vi "Formic Queen.vi"(8 "error in (no error)":errorcluster, 9 "SelfID":i32, 10 "Map":i32[](array[numeric]), 11 "Mother in":refnum<class "Mother.lvclass">) -> (0 "error out":errorcluster, 1 "Direction":T1, 2 "Action":T2, 3 "Mother out":refnum<class "Mother.lvclass">, 4 "Replicated Class":refnum<class "Mother.lvclass">)   [LabVIEW 2014, in "Mother.lvclass"]
uses:
  Mother.lvclass
  Action Enum.ctl
  Direction Enum.ctl
  Mother.lvclass/Mother.ctl
  SquareStatus.ctl
  Queen Bee Steps.ctl
  Formic Types.ctl
  SquareBattle.lvclass
panel:
  in  "Protectors":i32[](array[numeric])=[2, 6]
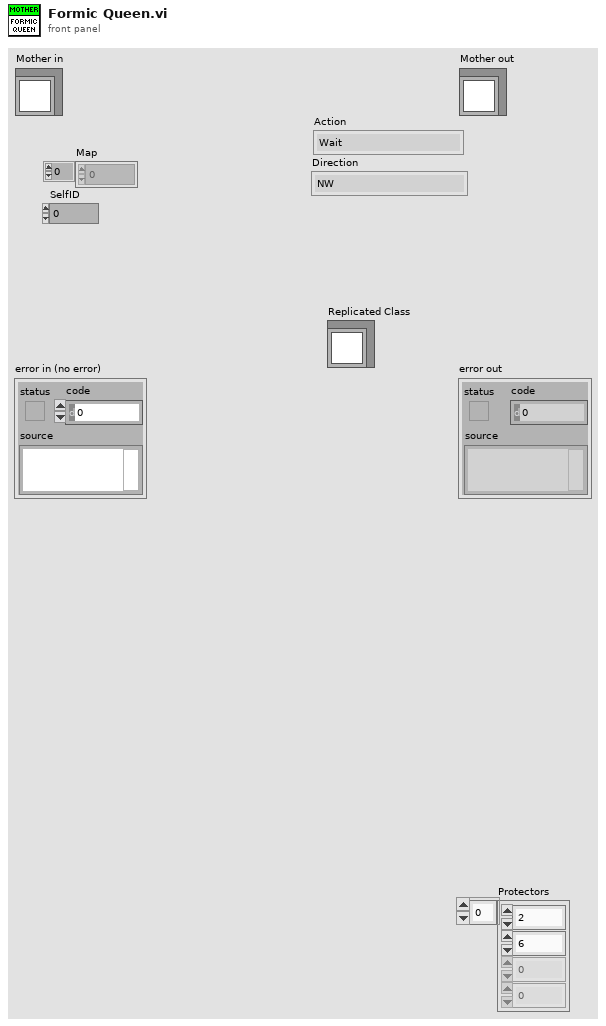
[diagram p1: front panel]
types:
  T1 = typedef "SquareBattle.lvclass/Direction Enum.ctl" = enum16{"NW", "N", "NE", "E", "SE", "S", "SW", "W"}
  T2 = typedef "SquareBattle.lvclass/Action Enum.ctl" = enum16{"Wait", "Move", "Attack", "Replicate"}
  T3 = typedef "Mother.lvclass/Formic Types.ctl" = enum16{"Queen Bee", "Protector Bee", "Daughter Bee", "Worker Bee", "Coward"}
  T4 = typedef "Mother.lvclass/SquareStatus.ctl" = cluster{"ID":i32, "Heartbeat":bool}
  T5 = typedef "Mother.lvclass/Queen Bee Steps.ctl" = enum16{"Attack?", "Migrate?", "Kamikaze?", "Protect?", "Procreate?", "Build Army"}
  T6 = typedef "Mother.lvclass/Kamikaze DVR.ctl" = refnum<data-value>
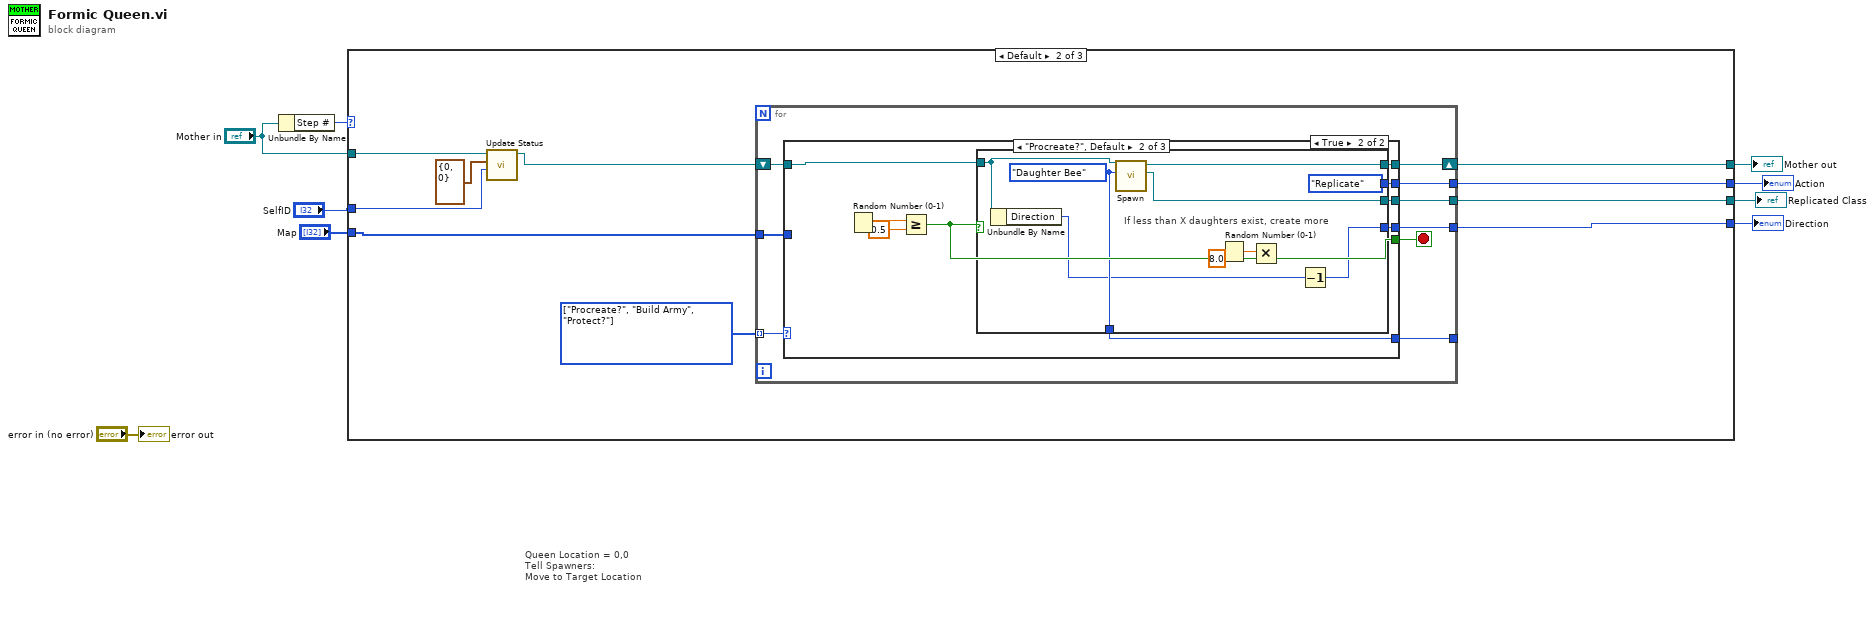
[diagram p0: block diagram]
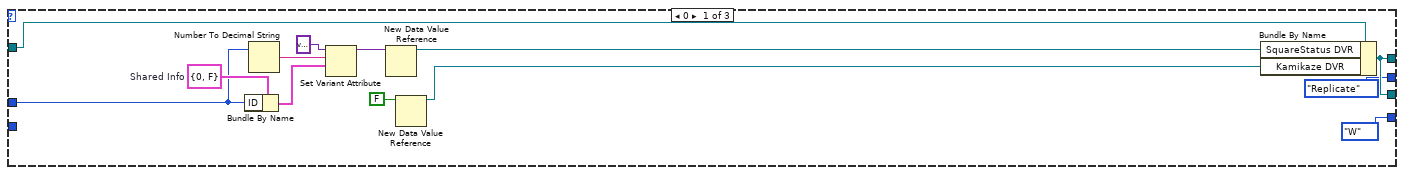
[diagram p2: hidden frame]
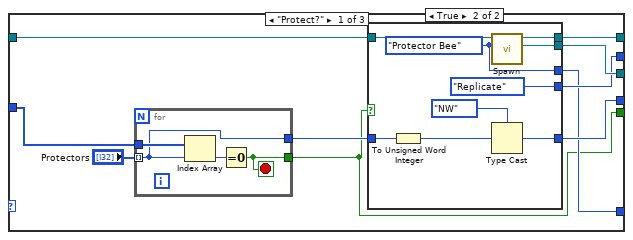
[diagram p3: hidden frame]
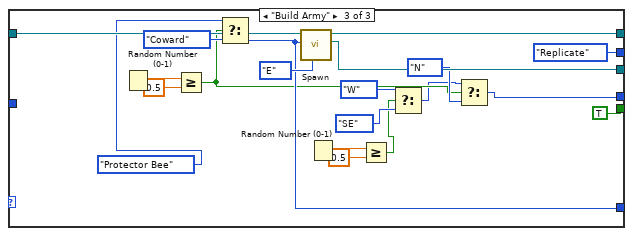
[diagram p6: hidden frame]
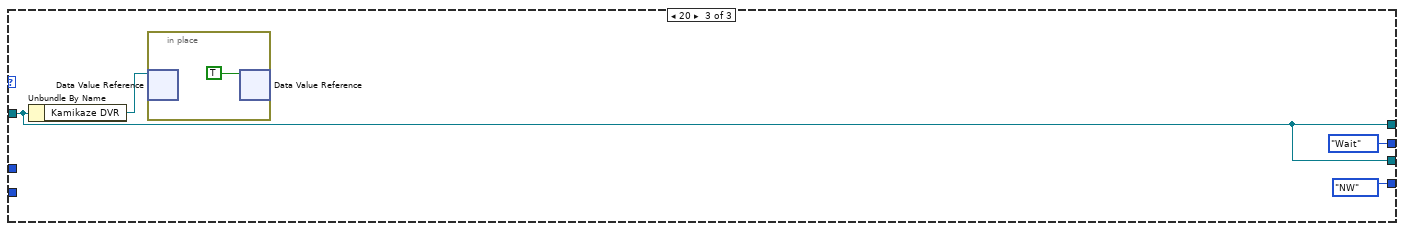
[diagram p7: hidden frame]
diagram:
  # "Queen Location = 0,0\nTell Spawners:\nMove to Target Location"
  n1 = Unbundle By Name("Mother in") -> ("Step #"=w6:i32)
  n2 = case shown="Default" w6 {
    tunnel: [w12 w28 w106] -> w8
    tunnel: "Mother in" -> [w14 w31 w106]
    tunnel: "SelfID" -> [w13 w30 _]
    tunnel: "Map" -> [_ w26 _]
    tunnel: [Action_Enum."Replicate" ("Action") w25 Action_Enum."Wait" ("Action")] -> w3
    tunnel: [Direction_Enum."W" ("Direction") w24 Direction_Enum."NW" ("Direction")] -> w2
    tunnel: [w12 w23 w106] -> w1
    frame 0 {
      w19 = T4 {"ID"=0, "Heartbeat"=FALSE}  # Shared Info
      n3 = Bundle By Name(cluster=w19, "ID"=w13) -> (w20:T4)
      n4 = Number To Decimal String(number=w13) -> (decimal integer string=w21:string)  [unwired: 1 in]
      n5 = Set Variant Attribute(Variant=variant ("variant"), name=w21, value=w20) -> (Variant out=w18:variant)  [unwired: 1 in, 2 out]
      n6 = New Data Value Reference(data value=w18) -> (data value reference=w17:refnum<data-value>)  [unwired: 1 in, 1 out]
      n7 = New Data Value Reference(data value=FALSE) -> (data value reference=w16:refnum<data-value>)  [unwired: 1 in, 1 out]
      n8 = Bundle By Name(cluster=w14, "SquareStatus DVR"=w17, "Kamikaze DVR"=w16) -> (w12:refnum<class "Mother.lvclass">)
    }
    frame Default {
      w27 = T5[] [enum."Procreate?", enum."Build Army", enum."Protect?"] items=["Attack?", "Migrate?", "Kamikaze?", "Protect?", "Procreate?", "Build Army"]
      n9 = call "Update Status.vi"("ID"=w30, "MyPosition"=cluster{"X":i32, "Y":i32} {"X"=0, "Y"=0}, "Mother in"=w31) -> ("Mother out"=w29:refnum<class "Mother.lvclass">)  [unwired: 8 in]
      n10 = for {
        shift-right: [w40] -> w28
        shift-left: w29 -> [w41]
        tunnel: [w39] -> w25
        tunnel: [w38] -> w24
        tunnel: w27 -> [w37] mode=indexing
        tunnel: [w35] -> w23
        tunnel: [w34] -> _
        tunnel: w26 -> [w33]
        stop <- w36 stop-if-true
        n11 = case shown="\"Procreate?\", Default" w37 {
          tunnel: w41 -> [w51 w69 w104]
          tunnel: [w50 w72 w101] -> w40
          tunnel: [w48 w74 Action_Enum."Replicate" ("Action")] -> w39
          tunnel: [w45 w73 w92] -> w38
          tunnel: [w43 w66 TRUE ("Enemy Found?")] -> w36
          tunnel: [w49 w71 w100] -> w35
          tunnel: [w44 w70 w94] -> w34
          tunnel: w33 -> [w42 _ _]
          frame "Protect?" {
            n12 = for {
              tunnel: w42 -> [w65]
              tunnel: [w64] -> w43
              tunnel: "Protectors" -> [w62] mode=indexing
              tunnel: [w62] -> w46
              stop <- w64 stop-if-true
              n13 = Index Array(array=w65, index=w62) -> (element=w63:i32)
              n14 = Equal To 0?(x=w63) -> (x = 0?=w64:bool)
            }
            n15 = case shown="True" w43 {
              tunnel: w51 -> [w52 w61]
              tunnel: [w52 w60] -> w50
              tunnel: [_ w59] -> w49
              tunnel: [_ Action_Enum."Replicate" ("Action")] -> w48
              tunnel: w46 -> [_ w56]
              tunnel: [_ w55] -> w45
              tunnel: [_ w53] -> w44
              frame False {
              }
              frame True {
                w53 = Formic_Types."Protector Bee"
                n16 = To Unsigned Word Integer(number=w56) -> (unsigned 16bit integer=w57:u16)
                n17 = call "Spawn.vi"(10:w53, "Mother in"=w61) -> ("Replicated Class"=w59:refnum<class "Mother.lvclass">, "Mother out"=w60:refnum<class "Mother.lvclass">)  [unwired: 7 in, 1 out]
                n18 = Type Cast(type=Direction_Enum."NW" ("Direction"), x=w57) -> (*(type *) &x=w55:T1)
              }
            }
          }
          frame "Procreate?", Default {
            n19 = Random Number (0-1)() -> (number: 0 to 1=w68:dbl)
            n20 = Greater Or Equal?(x=w68, y=0.5) -> (x >= y?=w66:bool)
            n21 = case shown="True" w66 {
              tunnel: [_ Action_Enum."Replicate" ("Action")] -> w74
              tunnel: [_ w78] -> w73
              tunnel: [w75 w83] -> w72
              tunnel: [_ w82] -> w71
              tunnel: [_ w81] -> w70
              tunnel: w69 -> [w75 w77]
              frame False {
              }
              frame True {
                w81 = Formic_Types."Daughter Bee"
                # "If less than X daughters exist, create more"
                n22 = Unbundle By Name(w77) -> ("Direction"=w76:T1)
                n23 = call "Spawn.vi"(10:w81, "Mother in"=w77) -> ("Replicated Class"=w82:refnum<class "Mother.lvclass">, "Mother out"=w83:refnum<class "Mother.lvclass">)  [unwired: 7 in, 1 out]
                n24 = Random Number (0-1)() -> (number: 0 to 1=w80:dbl)
                n25 = Multiply(x=w80, y=8.0) -> ()  [unwired: 1 out]
                n26 = Decrement(x=w76) -> (x-1=w78:T1)
              }
            }
          }
          frame "Build Army" {
            n27 = Random Number (0-1)() -> (number: 0 to 1=w95:dbl)
            n28 = Greater Or Equal?(x=w95, y=0.5) -> (x >= y?=w90:bool)
            n29 = Select(t=Formic_Types."Protector Bee", s=w90, f=Formic_Types."Coward") -> (s? t:f=w94:T3)
            n30 = call "Spawn.vi"("Start Direction"=Direction_Enum."E", 10:w94, "Mother in"=w104) -> ("Replicated Class"=w100:refnum<class "Mother.lvclass">, "Mother out"=w101:refnum<class "Mother.lvclass">)  [unwired: 6 in, 1 out]
            n31 = Random Number (0-1)() -> (number: 0 to 1=w89:dbl)
            n32 = Greater Or Equal?(x=w89, y=0.5) -> (x >= y?=w85:bool)
            n33 = Select(t=Direction_Enum."W", s=w85, f=Direction_Enum."SE" ("Direction")) -> (s? t:f=w87:T1)
            n34 = Select(t=w87, s=w90, f=Direction_Enum."N" ("Direction")) -> (s? t:f=w92:T1)
          }
        }
      }
    }
    frame 20 {
      n35 = Unbundle By Name(w106) -> ("Kamikaze DVR"=w108:T6)
      n36 = in-place {
        n37 = in-place-dvr #1(w108) -> ()  [unwired: 2 out]
        n38 = in-place-dvr #1(TRUE ("data value")) -> ()  [unwired: 2 out]
      }
    }
  }
  "Mother out" <- w8
  "Action" <- w3
  "Direction" <- w2
  "Replicated Class" <- w1
  "error out" <- "error in (no error)"
